vi "Set Button Enable States.vi"(8 "error in (no error)":errorcluster, 10 "Button States":T1, 11 "queue in":refnum<queue>) -> (0 "error out":errorcluster, 3 "queue out":refnum<queue>)   [LabVIEW 2010]
uses:
  RF Characterization States.ctl
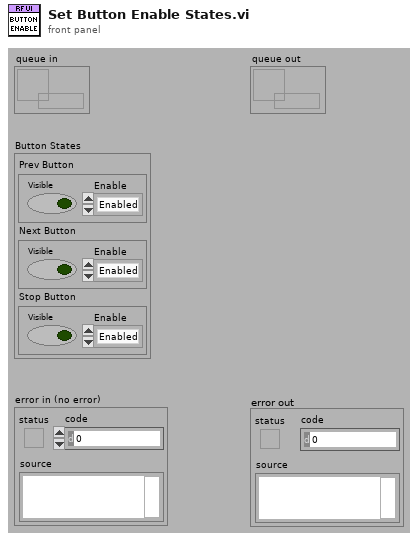
[diagram p1: front panel]
types:
  T1 = cluster{"Prev Button":cluster{"Visible":bool, "Enable":enum8{"Enabled", "Disabled", "Disabled and Grayed Out"}}, "Next Button":cluster{"Visible":bool, "Enable":enum8{"Enabled", "Disabled", "Disabled and Grayed Out"}}, "Stop Button":cluster{"Visible":bool, "Enable":enum8{"Enabled", "Disabled", "Disabled and Grayed Out"}}}
  T2 = typedef "RF Characterization States.ctl" = enum16{"Initialize", "Enable/Disable Navigation", "Set Next Action", "Set Prev Action", "Set Stop Action", "Prev Action Triggered", "Next Action Triggered", "Stop Action Triggered", "Move Gantry to Position", "Display Configuration Tab", "Check Configuration", "Display Attenuation Tab", "Check Attenuation Config", "Start Attenuation Test", "Check Attenuation Results", "Display Power Tab", "Check Power Config", "Start Power Test", "Check Power Results", "Display Mapping Tab", "Check Mapping Config", "Start Mapping Test", "Take Mapping Sample", "Finish Mapping Test", "Check Mapping Results", "Display Report Tab", "Generate Report", "Save Report", "Error", "Shutdown"}
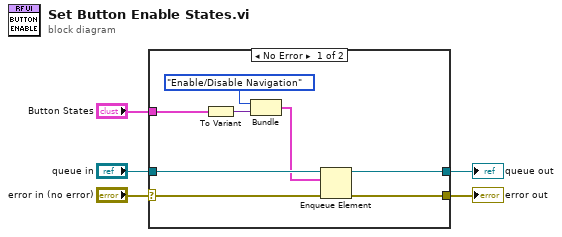
[diagram p0: block diagram]
diagram:
  n1 = case shown="No Error" "error in (no error)" {
    selector: "error in (no error)" -> [w6 w14]
    tunnel: "queue in" -> [w13 w15]
    tunnel: [w12 w15] -> w4
    tunnel: [w11 w14] -> w3
    tunnel: "Button States" -> [w8 _]
    frame No Error {
      n2 = To Variant(anything=w8) -> (Variant=w10:variant)
      n3 = Bundle("State"=RF_Characterization_States."Enable/Disable Navigation", "Variant"=w10) -> (w9:cluster{"State":T2, "Variant":variant})  [unwired: 1 in]
      n4 = Enqueue Element(queue=w13, element=w9, error in (no error)=w6) -> (queue out=w12:refnum<queue>, error out=w11:errorcluster)  [unwired: 1 in, 1 out]
    }
    frame Error {
    }
  }
  "queue out" <- w4
  "error out" <- w3
